vi "Result_Test.vi"(8 "error in (no error)":errorcluster caption="entrée d'erreur (pas d'erreur)", 11 "Get_Voltage en entrée":refnum<class "Zigbee_Network_Creator.lvclass">) -> (0 "error out":errorcluster caption="sortie d'erreur", 3 "Get_Voltage en sortie":refnum<class "Zigbee_Network_Creator.lvclass">)   [LabVIEW 2020, in "Library Test.lvlib" / "Zigbee_Network_Creator.lvclass"]
uses:
  Zigbee_Network_Creator.lvclass
  C:/Users/ngarcin/OneDrive - Altyor/Standard TB/Class/Test/Test (Default)/Test (Default).lvclass
  Zigbee_Send_Command_UART/Zigbee_Send_Command_UART.lvclass
  Zigbee_Network_Creator.lvclass/Zigbee_Network_Creator.ctl
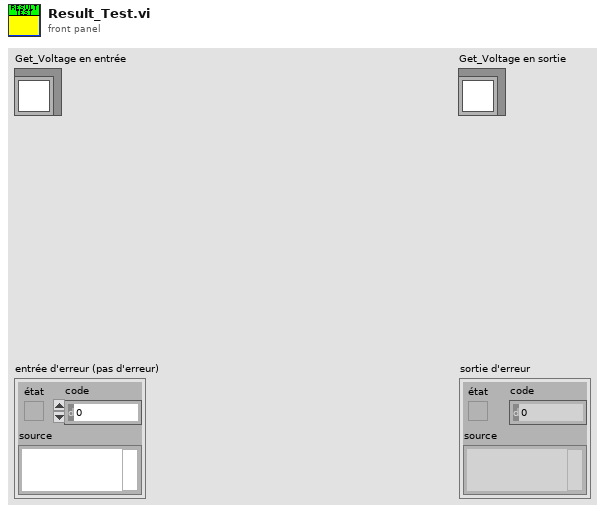
[diagram p1: front panel]
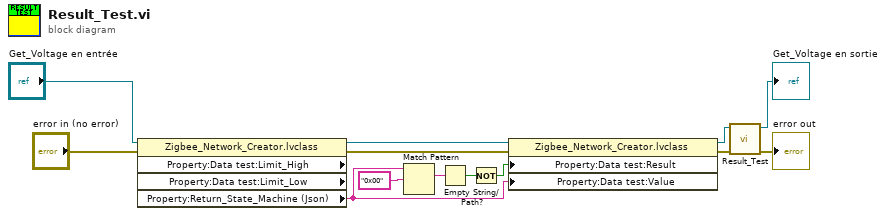
[diagram p0: block diagram]
diagram:
  n1 = property class="Zigbee_Network_Creator.lvclass" props=["Property:Data test:Limit_High", "Property:Data test:Limit_Low", "Property:Return_State_Machine (Json)"](reference="Get_Voltage en entrée", error in="error in (no error)") -> (reference out=w11:refnum<class "Zigbee_Network_Creator.lvclass">, error out=w10:errorcluster, "Property:Return_State_Machine (Json)"=w9:string)  [unwired: 2 out]
  n2 = Match Pattern(string=w9, regular expression="0x00" ("expression régulière")) -> (match substring=w8:string)  [unwired: 1 in, 3 out]
  n3 = Empty String/Path?(string/path=w8) -> (empty?=w7:bool)
  n4 = Not(x=w7) -> (.not. x?=w6:bool)
  n5 = property class="Zigbee_Network_Creator.lvclass"(reference=w11, error in=w10, "Property:Data test:Result"=w6, "Property:Data test:Value"=w9) -> (reference out=w3:refnum<class "Zigbee_Network_Creator.lvclass">, error out=w2:errorcluster)
  n6 = call-parent "Result_Test.vi"("error in (no error)"=w2, "Get_Voltage en entrée"=w3) -> ("error out"=→"error out":errorcluster, "Get_Voltage en sortie"=→"Get_Voltage en sortie":refnum<class "Zigbee_Network_Creator.lvclass">)  [unwired: 8 in]
